vi "Stop ext modules.vi"(8 "error in":errorcluster) -> (0 "error out":errorcluster)   [LabVIEW 2023, in "Dispatcher.lvlib"]
uses:
  Dispatcher.lvlib
  Graph_data_collector/Graph_data_collector.lvlib
  Registration/Registration.lvlib
  Initial Data/Initial Data.lvlib
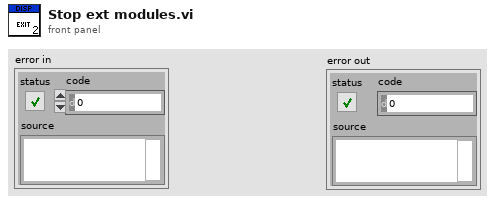
[diagram p1: front panel]
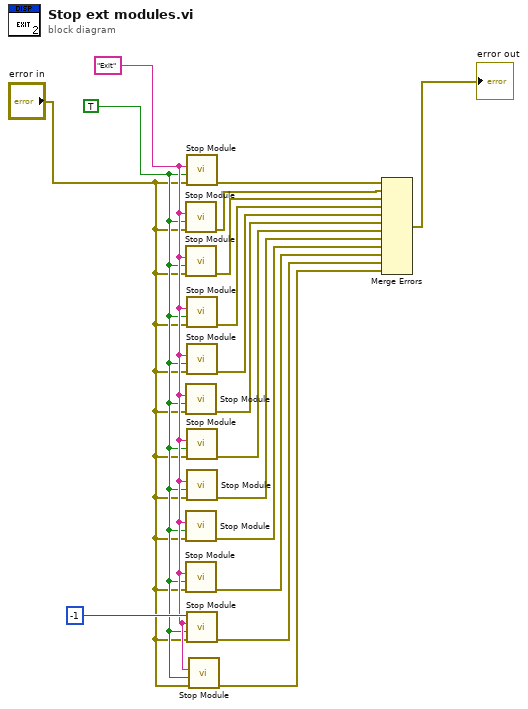
[diagram p0: block diagram]
diagram:
  w4 = "Exit" ("Origin")
  w3 = TRUE ("Wait for Module to Stop? (F)")
  n1 = call "Stop Module.vi"("error in"="error in", "Wait for Module to Stop? (F)"=w3, "Origin"=w4) -> ("error out"=w15:errorcluster)  [unwired: 8 in]
  n2 = call "Stop Module.vi"("error in"="error in", "Wait for Module to Stop? (F)"=w3, "Origin"=w4) -> ("error out"=w14:errorcluster)  [unwired: 8 in]
  n3 = call "Stop Module.vi"("error in"="error in", "Wait for Module to Stop? (F)"=w3, "Origin"=w4) -> ("error out"=w11:errorcluster)  [unwired: 8 in]
  n4 = call "Stop Module.vi"("error in"="error in", "Wait for Module to Stop? (F)"=w3, "Origin"=w4) -> ("error out"=w8:errorcluster)  [unwired: 8 in]
  n5 = call "Stop Module.vi"("error in"="error in", "Wait for Module to Stop? (F)"=w3, "Origin"=w4) -> ("error out"=w7:errorcluster)  [unwired: 8 in]
  n6 = call "Stop Module.vi"("error in"="error in", "Wait for Module to Stop? (F)"=w3, "Origin"=w4) -> ("error out"=w17:errorcluster)  [unwired: 8 in]
  n7 = call "Stop Module.vi"("error in"="error in", "Wait for Module to Stop? (F)"=w3, "Origin"=w4) -> ("error out"=w13:errorcluster)  [unwired: 8 in]
  n8 = call "Stop Module.vi"("error in"="error in", "Wait for Module to Stop? (F)"=w3, "Origin"=w4) -> ("error out"=w12:errorcluster)  [unwired: 8 in]
  n9 = call "Stop Module.vi"("error in"="error in", "Wait for Module to Stop? (F)"=w3, "Origin"=w4) -> ("error out"=w10:errorcluster)  [unwired: 8 in]
  n10 = call "Stop Module.vi"("error in"="error in", "Wait for Module to Stop? (F)"=w3, "Origin"=w4) -> ("error out"=w9:errorcluster)  [unwired: 8 in]
  n11 = call "Stop Module.vi"("error in"="error in", "Wait for Module to stop? (F)"=w3, "Origin"=w4, "Module ID"=-1) -> ("error out"=w5:errorcluster)  [unwired: 7 in]
  n12 = call "Stop Module.vi"("error in"="error in", "Wait for Module to Stop? (F)"=w3, "Origin"=w4) -> ("error out"=w1:errorcluster)  [unwired: 8 in]
  n13 = Merge Errors(w17, w15, w14, w13, w12, w11, w10, w9, w8, w7, w5, w1) -> (→"error out":errorcluster)
